vi "Died.vi"(8 "error in (no error)":errorcluster, 9 "Y":i32, 10 "X":i32, 11 "TurnProcessor in":refnum<class "TurnProcessor.lvclass">) -> (0 "error out":errorcluster, 3 "TurnProcessor out":refnum<class "TurnProcessor.lvclass">)   [LabVIEW 2015, in "Experience.lvlib" / "TurnProcessor.lvclass"]
uses:
  TurnProcessor.lvclass
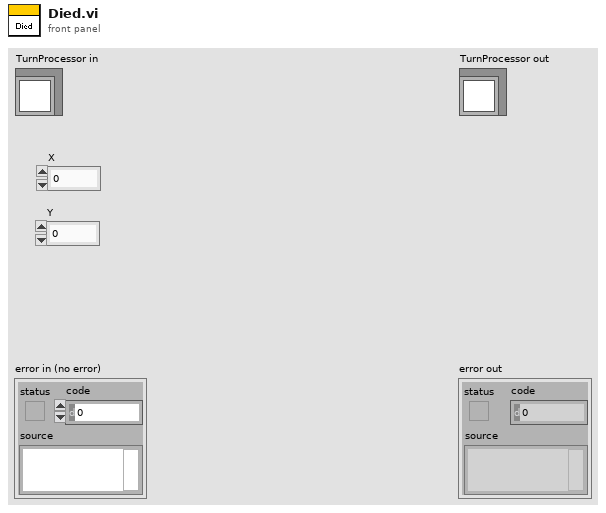
[diagram p1: front panel]
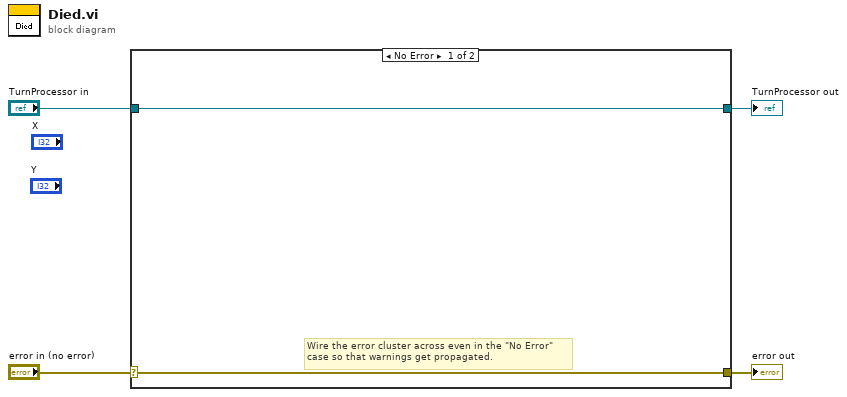
[diagram p0: block diagram]
diagram:
  n1 = case shown="No Error" "error in (no error)" {
    selector: "error in (no error)" -> [w5 w8]
    tunnel: [w5 w8] -> w3
    tunnel: [w6 w7] -> w1
    tunnel: "TurnProcessor in" -> [w6 w7]
    frame No Error {
      # "Wire the error cluster across even in the \"No Error\"\ncase so that warnings get propagated."
    }
    frame Error {
    }
  }
  "error out" <- w3
  "TurnProcessor out" <- w1
